vi "Auto selection sub.vi"() -> ()   [LabVIEW 2017, in "labview-standard-library.lvlib"]
uses:
  labview-standard-library.lvlib
panel:
  out "NT var: current file name":string
  in  "Use this auto?":bool
  in  "stop":bool
  in  "Select auto mode":i32(listbox)
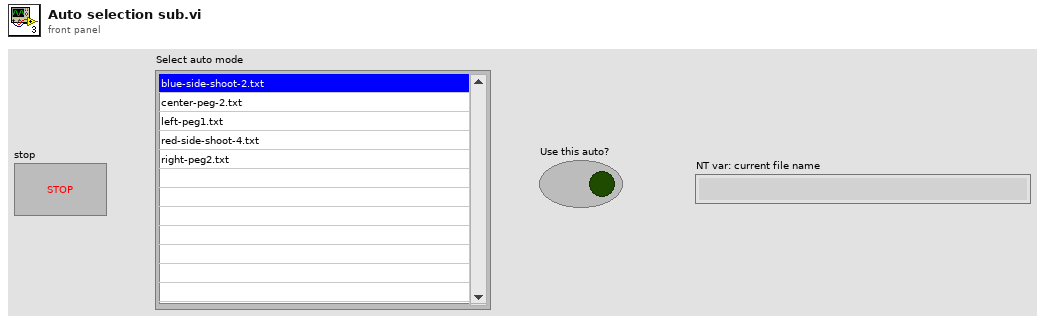
[diagram p1: front panel]
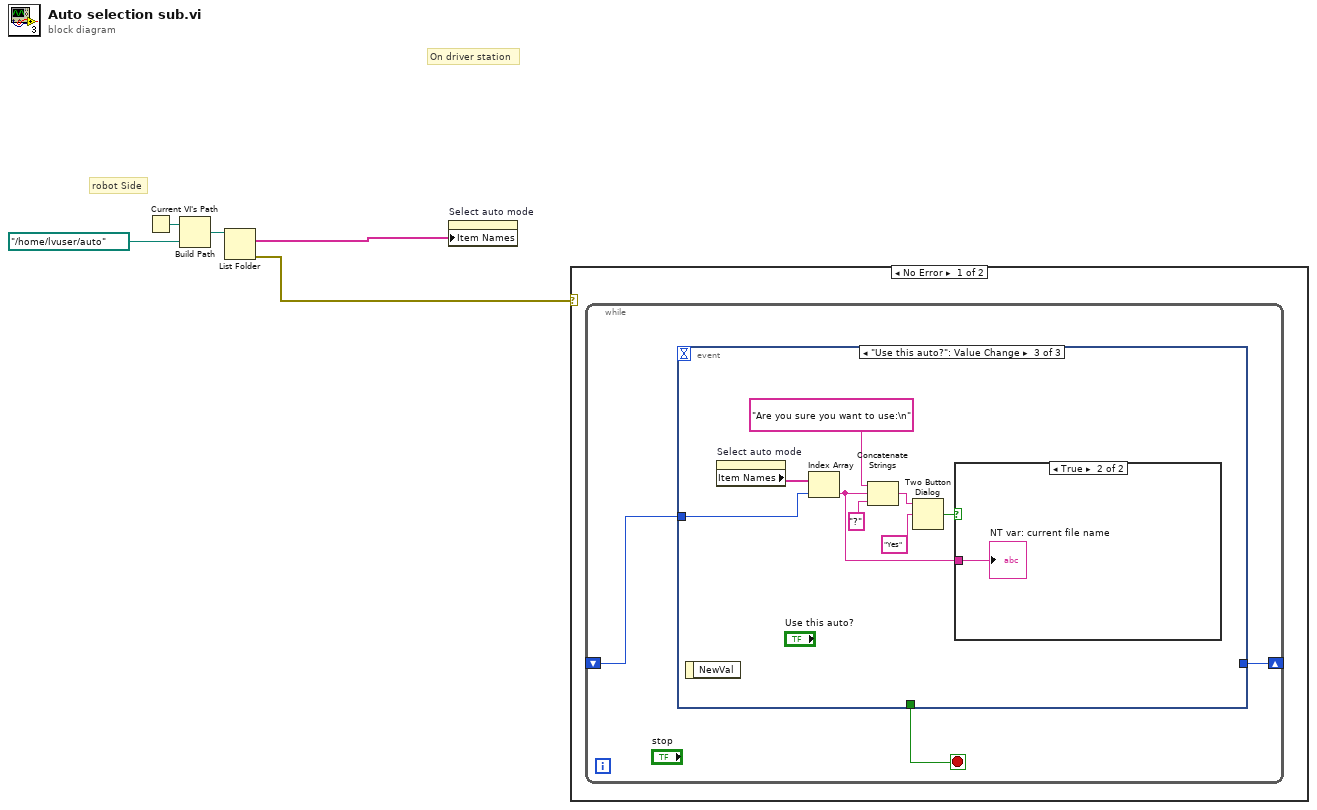
[diagram p0: block diagram]
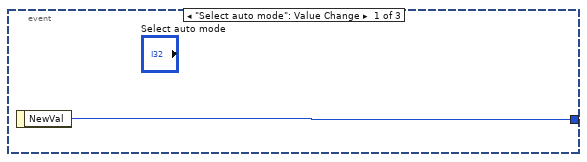
[diagram p2: hidden frame]
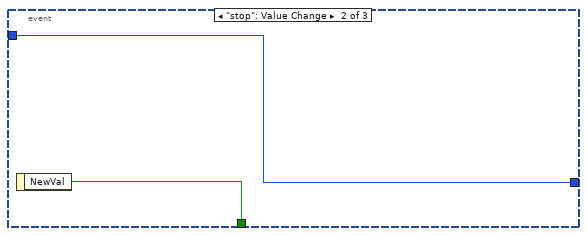
[diagram p3: hidden frame]
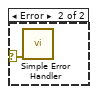
[diagram p5: hidden frame]
diagram:
  # "robot Side"
  # "On driver station"
  n1 = Current VI's Path() -> (path=w5:path)
  n2 = Build Path(base path=w5, name or relative path=path "../home/lvuser/auto") -> (appended path=w4:path)
  n3 = List Folder(path=w4) -> (filenames=w3:string[], error out=w2:errorcluster)  [unwired: 3 in, 2 out]
  n4 = property on="Select auto mode" class="LstBox (strict)"("Item Names"=w3) -> ()  [unwired: 2 in, 2 out]
  n5 = case shown="No Error" w2 {
    selector: w2 -> [_ w21]
    frame No Error {
      n6 = while {
        shift-right: [w7] -> _
        shift-left: _ -> [w6]
        stop <- w8 stop-if-true
        n7 = event shown="[2] \"Use this auto?\": Value Change" {
          selector: _ -> [_ _ _]
          dyn-events: _ -> [_ _ _]
          timeout: _ -> [_ _ _]
          tunnel: [_ w11 _] -> w8
          tunnel: [w9 w10 _] -> w7
          tunnel: w6 -> [_ w10 w19]
          event "Select auto mode": Value Change {
            n8 = event-data() -> ("NewVal"=w9:i32)  [unwired: 1 in]
          }
          event "stop": Value Change {
            n9 = event-data() -> ("NewVal"=w11:bool)  [unwired: 1 in]
          }
          event "Use this auto?": Value Change {
            n10 = event-data() -> ()  [unwired: 1 in, 1 out]
            n11 = property on="Select auto mode" class="LstBox (strict)"() -> ("Item Names"=w17:string[])  [unwired: 2 in, 2 out]
            n12 = Index Array(array=w17, index=w19) -> (element=w13:string)
            n13 = Concatenate Strings("Are you sure you want to use:\n" ("message"), w13, "?") -> (w15:string)
            n14 = Two Button Dialog(message=w15, 2:"Yes" ("T button name (\"OK\")")) -> (T button?=w14:bool)  [unwired: 1 in]
            n15 = case shown="True" w14 {
              tunnel: w13 -> [_ w20]
              frame False {
              }
              frame True {
                "NT var: current file name" <- w20
              }
            }
          }
        }
      }
    }
    frame Error {
      n16 = call <vilib>:"Simple Error Handler.vi"("error in (no error)"=w21) -> ()  [unwired: 4 in, 5 out]
    }
  }
